vi "DisplayScanPlane.vi"(6 "Header":T2, 7 "Frame Duration (ms)":u32=100, 8 "error in (no error)":errorcluster, 10 "PMT Channel":i32, 11 "Scan Data":dbl[][][][](array[numeric])) -> (0 "error out":errorcluster)   [LabVIEW 2011]
panel:
  out "Image":T1(plugin-control)
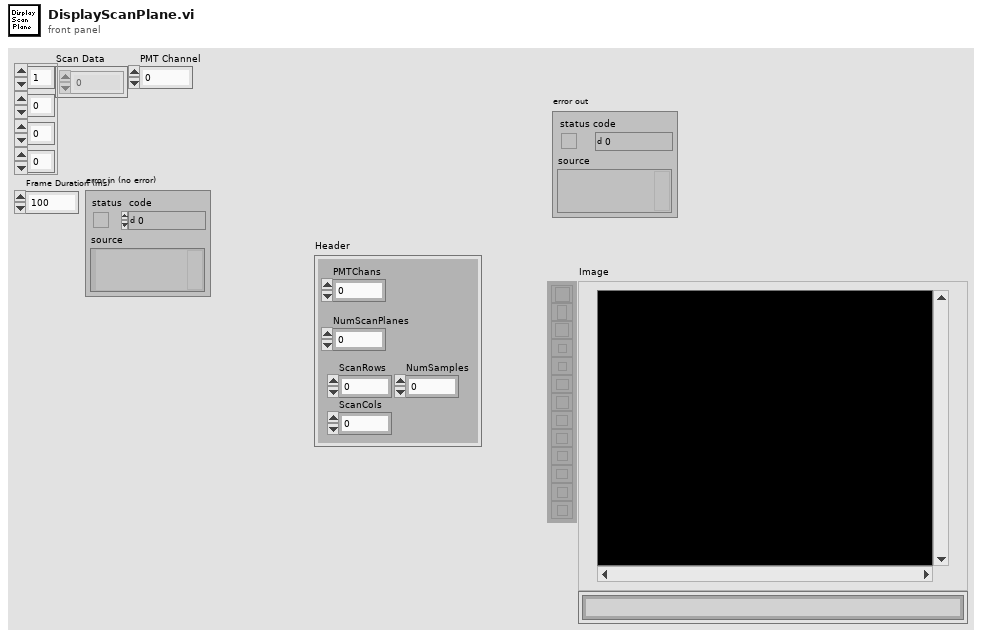
[diagram p1: front panel]
types:
  T1 = typedef "IMAQ Image.ctl" = refnum<image>
  T2 = cluster{"PMTChans":i32, "NumScanPlanes":i32, "ScanRows":i32, "ScanCols":i32, "NumSamples":i32}
  T3 = typedef "Image Type" = u32
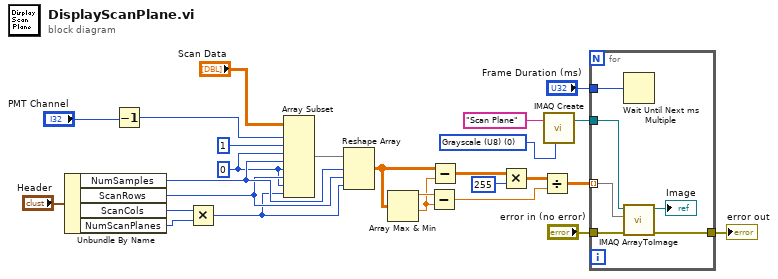
[diagram p0: block diagram]
diagram:
  w15 = T3 0 items=["Grayscale (U8)", "Grayscale (I16)", "Grayscale (SGL)", "Complex (CSG)", "RGB (U32)", "HSL (U32)", "RGB (U64)", "Grayscale (U16)"] ("Image Type")
  w6 = 0 ("index")
  n1 = Unbundle By Name("Header") -> ("NumSamples"=w13:i32, "ScanRows"=w12:i32, "ScanCols"=w5:i32, "NumScanPlanes"=w4:i32)
  n2 = Decrement(x="PMT Channel") -> (x-1=w1:i32)
  n3 = Multiply(x=w5, y=w4) -> (x*y=w3:i32)
  n4 = Array Subset(array="Scan Data", index (dim 0)=w1, length (dim 0)=1 ("length"), index (dim 1)=w6, length (dim 1)=w13, index (dim 2)=w6, length (dim 2)=w12, index (dim 3)=w6, length (dim 3)=w3) -> (w26:dbl[][][][])
  n5 = Reshape Array(w26, w13, w12, w3) -> (w24:dbl[][][])
  n6 = Array Max & Min(array=w24) -> (max value=w25:dbl, min value=w23:dbl)  [unwired: 2 out]
  n7 = Subtract(x=w25, y=w23) -> (x-y=w19:dbl)
  n8 = Subtract(x=w24, y=w23) -> (x-y=w22:dbl[][][])
  n9 = Multiply(x=w22, y=255) -> (x*y=w20:dbl[][][])
  n10 = Divide(x=w20, y=w19) -> (x/y=w18:dbl[][][])
  n11 = call "IMAQ Create"("Image Name"="Scan Plane", "Image Type"=w15) -> ("New Image"=w17:T1)  [unwired: 3 in, 1 out]
  n12 = for {
    tunnel: w18 -> [w32] mode=indexing
    tunnel: w17 -> [w31]
    tunnel: "Frame Duration (ms)" -> [w30]
    tunnel: "error in (no error)" -> [w29]
    tunnel: [w28] -> w7
    n13 = Wait Until Next ms Multiple(millisecond multiple=w30) -> ()  [unwired: 1 out]
    n14 = call "IMAQ ArrayToImage"("error in (no error)"=w29, "Image Pixels (U8)"=w32, "Image"=w31) -> ("error out"=w28:errorcluster, "Image Out"=→"Image":T1)  [unwired: 7 in]
  }
  "error out" <- w7
